vi "Create Index Job File.vi"(0 "job file location":path, 5 "paths to be indexed":path[](array[path]), 7 "path type (files)":enum16{"files", "folders"}(ring), 11 "error in (no error)":errorcluster) -> (4 "job file location out":path, 15 "error out":errorcluster)   [LabVIEW 2020, in "NI_DataFinder.lvlib"]
doc: "Creates a job file for indexing certain files or folders from the search areas of a DataFinder server."
uses:
  <vilib>/DataFinder/NI_DataFinder.lvlib
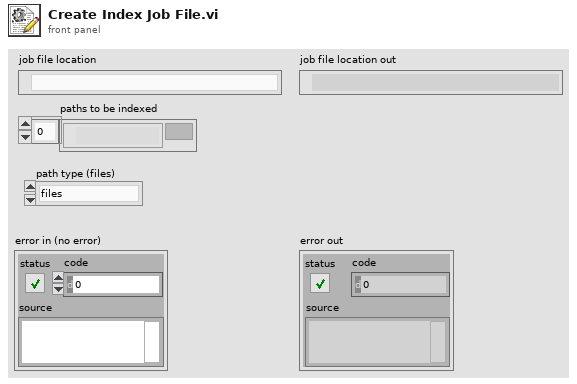
[diagram p1: front panel]
types:
  T1 = enum16{"open", "replace", "create", "open or create", "replace or create", "replace or create with confirmation"}
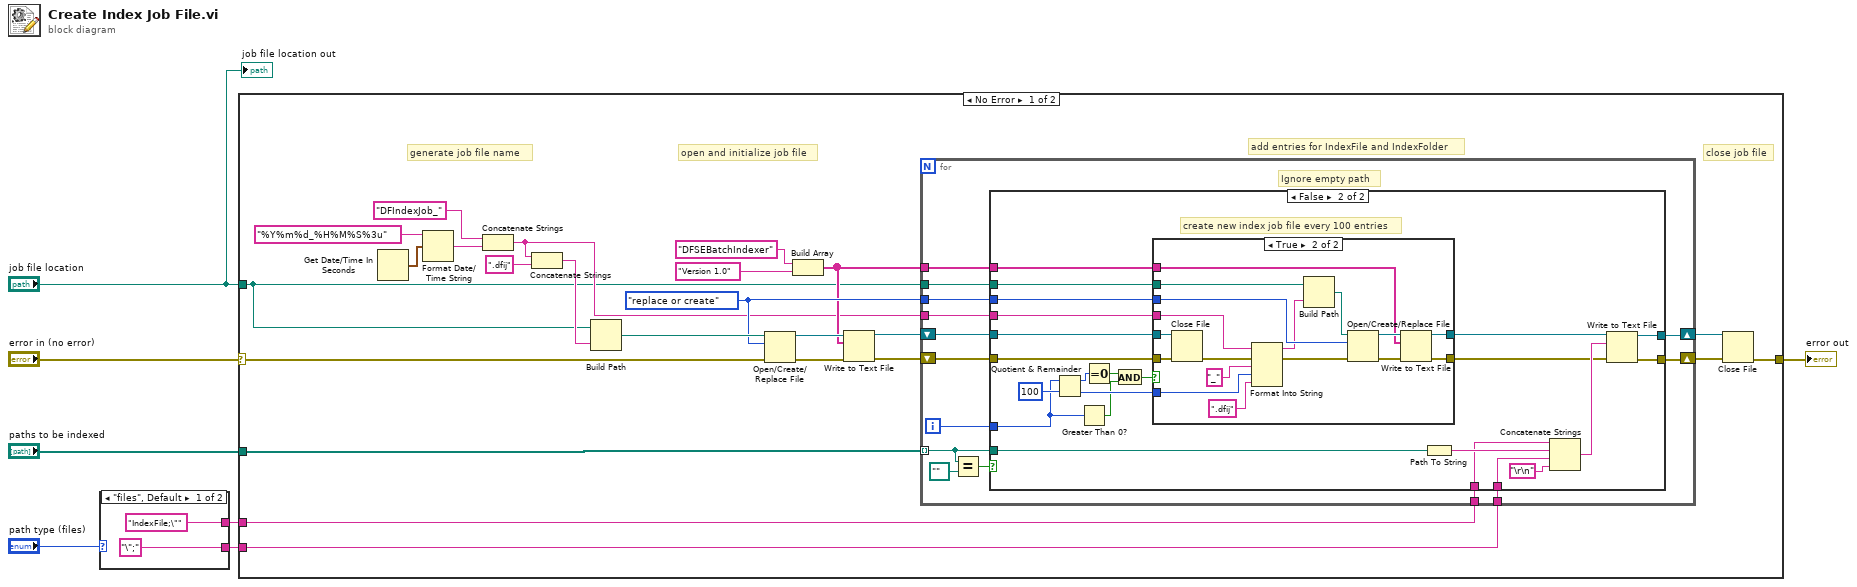
[diagram p0: block diagram]
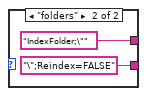
[diagram p2: hidden frame]
diagram:
  n1 = case shown="\"files\", Default" "path type (files)" {
    tunnel: ["IndexFile;\"" "IndexFolder;\""] -> w2
    tunnel: ["\";" "\";Reindex=FALSE"] -> w1
    frame "files", Default {
    }
    frame "folders" {
    }
  }
  n2 = case shown="No Error" "error in (no error)" {
    selector: "error in (no error)" -> [w27 w94]
    tunnel: [w26 w94] -> w6
    tunnel: "paths to be indexed" -> [w23 _]
    tunnel: "job file location" -> [w14 _]
    tunnel: w2 -> [w13 _]
    tunnel: w1 -> [w12 _]
    frame No Error {
      w20 = T1."replace or create" ("operation (0:open)")
      # "close job file"
      # "add entries for IndexFile and IndexFolder"
      # "open and initialize job file"
      # "generate job file name"
      n3 = Get Date/Time In Seconds() -> (seconds since 1Jan1904=w35:timestamp)
      n4 = Format Date/Time String(time format string (%c)="%Y%m%d_%H%M%S%3u", seconds (now)=w35) -> (date/time string=w16:string)  [unwired: 1 in]
      n5 = Concatenate Strings("DFIndexJob_", w16) -> (w15:string)
      n6 = Concatenate Strings(w15, ".dfij") -> (w18:string)
      n7 = Build Path(base path=w14, name or relative path=w18) -> (appended path=w32:path)
      n8 = Open/Create/Replace File(file path (use dialog)=w32, error in=w27, operation (0:open)=w20) -> (refnum out=w29:refnum<file>, error out=w28:errorcluster)  [unwired: 3 in, 1 out]
      n9 = Build Array("DFSEBatchIndexer", "Version 1.0") -> (w19:string[])
      n10 = Write to Text File(file (use dialog)=w29, text=w19, error in=w28) -> (refnum out=w22:refnum<file>, error out=w25:errorcluster)  [unwired: 1 in, 1 out]
      n11 = for {
        shift-right: [w49] -> w24
        shift-left: w25 -> [w46]
        tunnel: w23 -> [w36] mode=indexing
        shift-right: [w48] -> w21
        shift-left: w22 -> [w47]
        tunnel: w20 -> [w45]
        tunnel: w19 -> [w44]
        tunnel: w15 -> [w43]
        tunnel: w14 -> [w42]
        tunnel: w13 -> [w40]
        tunnel: w12 -> [w39]
        i -> [w41]
        # "Ignore empty path"
        n12 = Equal?(x=w36, y=path "") -> (x = y?=w38:bool)
        n13 = case shown="False" w38 {
          tunnel: [w50 w74] -> w49
          tunnel: [w51 w71] -> w48
          tunnel: w47 -> [w51 w69]
          tunnel: w46 -> [w50 w67]
          tunnel: w45 -> [_ w66]
          tunnel: w44 -> [_ w65]
          tunnel: w43 -> [_ w64]
          tunnel: w42 -> [_ w61]
          tunnel: w41 -> [_ w60]
          tunnel: w36 -> [_ w55]
          tunnel: w40 -> [_ w53]
          tunnel: w39 -> [_ w52]
          frame True {
          }
          frame False {
            # "create new index job file every 100 entries"
            n14 = Quotient & Remainder(x=w60, y=100) -> (x-y*floor(x/y)=w57:i32, floor(x/y)=w63:i32)
            n15 = Greater Than 0?(x=w60) -> (x > 0?=w59:bool)
            n16 = Equal To 0?(x=w57) -> (x = 0?=w56:bool)
            n17 = And(x=w56, y=w59) -> (x .and. y?=w58:bool)
            n18 = case shown="True" w58 {
              tunnel: w69 -> [w76 w92]
              tunnel: [w76 w87] -> w68
              tunnel: w67 -> [w75 w93]
              tunnel: [w75 w90] -> w54
              tunnel: w66 -> [_ w91]
              tunnel: w65 -> [_ w86]
              tunnel: w63 -> [_ w83]
              tunnel: w64 -> [_ w77]
              tunnel: w61 -> [_ w80]
              frame False {
              }
              frame True {
                n19 = Close File(refnum=w92, error in=w93) -> (error out=w85:errorcluster)  [unwired: 1 out]
                n20 = Format Into String(initial string=w77, error in=w85, "_", w83, ".dfij") -> (resulting string=w79:string, error out=w84:errorcluster)  [unwired: 1 in]
                n21 = Build Path(base path=w80, name or relative path=w79) -> (appended path=w78:path)
                n22 = Open/Create/Replace File(file path (use dialog)=w78, error in=w84, operation (0:open)=w91) -> (refnum out=w88:refnum<file>, error out=w89:errorcluster)  [unwired: 3 in, 1 out]
                n23 = Write to Text File(file (use dialog)=w88, text=w86, error in=w89) -> (refnum out=w87:refnum<file>, error out=w90:errorcluster)  [unwired: 1 in, 1 out]
              }
            }
            n24 = Path To String(path=w55) -> (string=w73:string)
            n25 = Concatenate Strings(w53, w73, w52, "\r\n") -> (w72:string)
            n26 = Write to Text File(file (use dialog)=w68, text=w72, error in=w54) -> (refnum out=w71:refnum<file>, error out=w74:errorcluster)  [unwired: 1 in, 1 out]
          }
        }
      }
      n27 = Close File(refnum=w21, error in=w24) -> (error out=w26:errorcluster)  [unwired: 1 out]
    }
    frame Error {
    }
  }
  "error out" <- w6
  "job file location out" <- "job file location"
